vi "Find All By Key.vi"(8 "error in":errorcluster, 10 "Key":string, 11 "Fast Tree in":refnum<class "Fast Tree.lvclass">) -> (0 "error out":errorcluster, 2 "Found Items":T1(array[cluster]), 3 "Fast Tree out":refnum<class "Fast Tree.lvclass">)   [LabVIEW 2019, in "Fast Tree.lvclass"]
uses:
  Fast Tree.lvclass
  Fast Tree.lvclass/Fast Tree.ctl
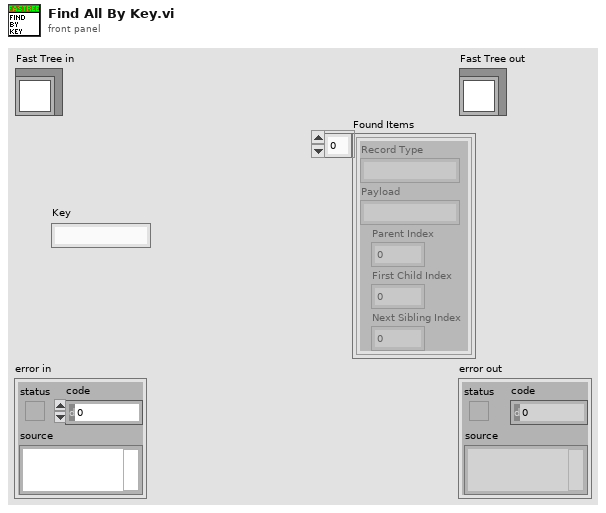
[diagram p1: front panel]
types:
  T1 = cluster{"Record Type":string, "Payload":string, "Parent Index":i32, "First Child Index":i32, "Next Sibling Index":i32}[]
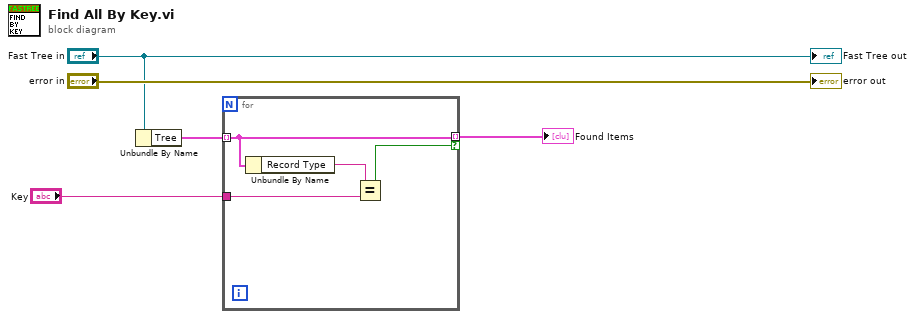
[diagram p0: block diagram]
diagram:
  n1 = Unbundle By Name("Fast Tree in") -> ("Tree"=w3:T1)
  n2 = for {
    tunnel: w3 -> [w7] mode=indexing
    tunnel: "Key" -> [w9]
    tunnel: [w7] -> w1 mode=indexing if=w6
    n3 = Unbundle By Name(w7) -> ("Record Type"=w8:string)
    n4 = Equal?(x=w8, y=w9) -> (x = y?=w6:bool)
  }
  "Found Items" <- w1
  "error out" <- "error in"
  "Fast Tree out" <- "Fast Tree in"
